vi "Init.vi"(8 "error in (no error)":errorcluster, 11 "Scene Collection Name":string) -> (0 "error out":errorcluster, 3 "CreateSceneCollection out":refnum<class "CreateSceneCollection.lvclass">)   [LabVIEW 2020, in "obs-websocket.lvlib" / "CreateSceneCollection.lvclass"]
uses:
  CreateSceneCollection.lvclass
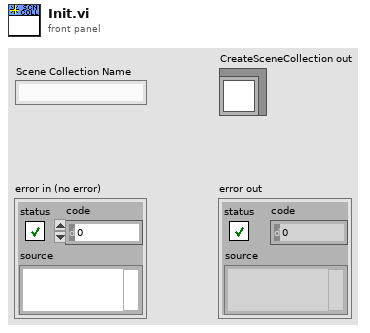
[diagram p1: front panel]
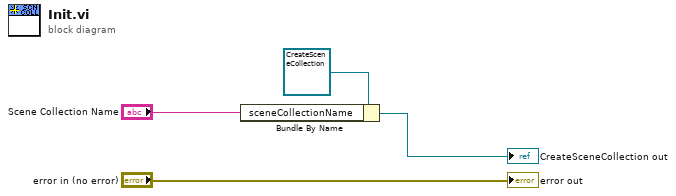
[diagram p0: block diagram]
diagram:
  n1 = Bundle By Name(cluster=refnum<class "CreateSceneCollection.lvclass"> refnum ("CreateSceneCollection in"), "sceneCollectionName"="Scene Collection Name") -> (→"CreateSceneCollection out":refnum<class "CreateSceneCollection.lvclass">)
  "error out" <- "error in (no error)"
